vi "Stream to Text File - 1 channel 1 sample.vi"() -> ()   [LabVIEW 2020]
uses:
  <vilib>/DAQmx/read.llb/DAQmx Read (Analog DBL 1Chan 1Samp).vi
  <vilib>/DAQmx/create/channels.llb/DAQmx Create Channel (AI-Temperature-Thermocouple).vi
  <vilib>/DAQmx/configure/timing.llb/DAQmx Timing (Sample Clock).vi
  <vilib>/DAQmx/miscellaneous.llb/DAQmx Fill In Error Info.vi
panel:
  in  "maximum value":dbl=100.0
  in  "minimum value":dbl
  in  "Thermocouple Channel":tag="PCI-6221/ai1"
  in  "stop":bool
  out "Waveform Chart":dbl(graph)=61.68840446814595
  # "Measurement Range"
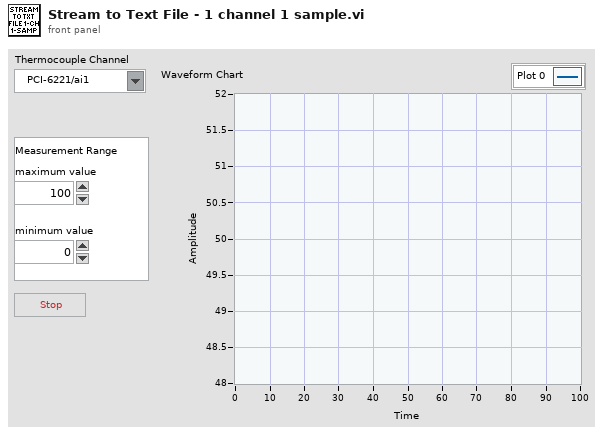
[diagram p1: front panel]
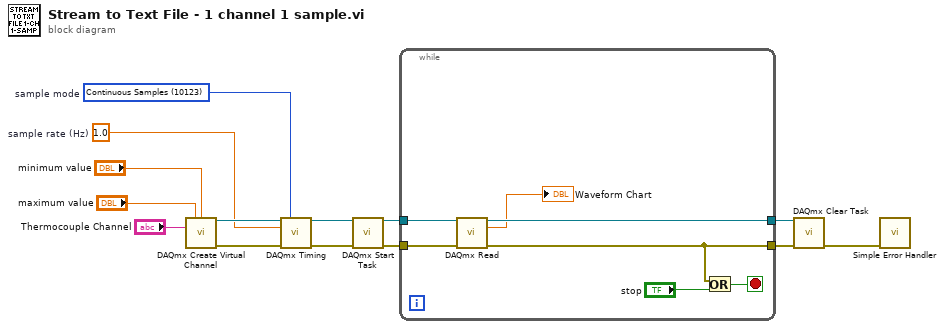
[diagram p0: block diagram]
diagram:
  w9 = 1.0  # sample rate (Hz)
  w10 = 10123 items=["Finite Samples"=10178, "Continuous Samples"=10123, "Hardware Timed Single Point"=12522]  # sample mode
  n1 = call-poly <vilib>:"DAQmx Create Virtual Channel.vi"("maximum value"="maximum value", "minimum value"="minimum value", "physical channels"="Thermocouple Channel") -> ("task out"=w14:refnum<k21>, "error out"=w13:errorcluster)  [unwired: 11 in]
  n2 = call-poly <vilib>:"DAQmx Timing.vi"("task/channels in"=w14, "sample mode"=w10, "rate"=w9, "error in"=w13) -> ("task out"=w8:refnum<k21>, "error out"=w7:errorcluster)  [unwired: 10 in]
  n3 = call <vilib>:"DAQmx Start Task.vi"("task/channels in"=w8, "error in"=w7) -> ("task out"=w12:refnum<k21>, "error out"=w11:errorcluster)  [unwired: 12 in]
  n4 = while {
    tunnel: w12 -> [w21]
    tunnel: w11 -> [w20]
    tunnel: [w19] -> w6
    tunnel: [w15] -> w2
    stop <- w18 stop-if-true
    n5 = call-poly <vilib>:"DAQmx Read.vi"("task/channels in"=w21, "error in"=w20) -> ("task out"=w19:refnum<k21>, "data"=→"Waveform Chart":dbl, "error out"=w15:errorcluster)  [unwired: 11 in]
    n6 = Or(x=w15, y="stop") -> (x .or. y?=w18:bool)
  }
  n7 = call <vilib>:"DAQmx Clear Task.vi"("task in"=w6, "error in"=w2) -> ("error out"=w1:errorcluster)  [unwired: 13 in]
  n8 = call <vilib>:"Simple Error Handler.vi"("error in (no error)"=w1) -> ()  [unwired: 4 in, 5 out]
